vi "Configure Aperture.vi"(8 "error in (no error)":errorcluster, 9 "Aperture Time (1: 1s)":dbl(ring)=1.0 items=["1s"=1.0, "100ms"=0.1], 10 "Display (0: Primary Display)":i32(ring) items=["Primary Display", "Secondary Display"], 11 "VISA resource name":refnum<visa-resource-name>) -> (0 "error out":errorcluster, 3 "VISA resource name out":refnum<visa-resource-name>)   [LabVIEW 2020, in "Agilent 34405.lvlib"]
doc: "Configures the aperture time (also called gate time) for frequency measurements.\n\n<B>Notes:</B>\n(1) This VI affects the <B>Frequency</B> measurements only. \n(2) This VI only support <B>Agilent 34450A</B>."
uses:
  <instrlib>/Agilent 34405/Agilent 34405.lvlib
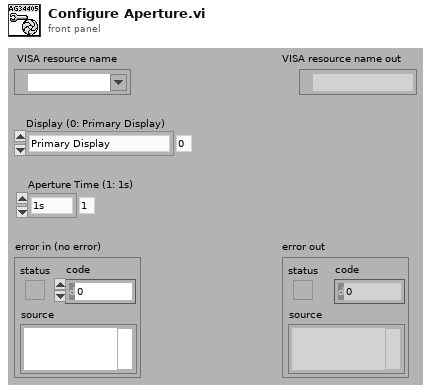
[diagram p1: front panel]
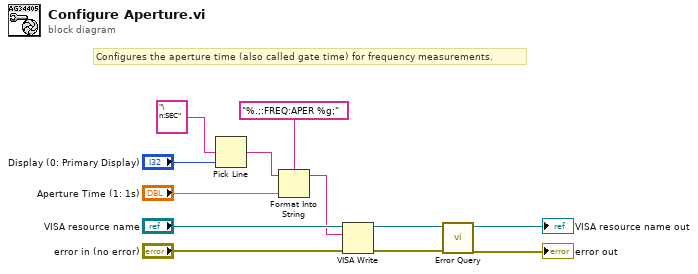
[diagram p0: block diagram]
diagram:
  # "Configures the aperture time (also called gate time) for frequency measurements."
  n1 = Pick Line(multi-line string="\n:SEC", line index="Display (0: Primary Display)") -> (output string=w1:string)  [unwired: 1 out]
  n2 = Format Into String(format string="%.;:FREQ:APER %g;", initial string=w1, "Aperture Time (1: 1s)") -> (resulting string=w3:string)  [unwired: 1 in, 1 out]
  n3 = VISA Write(VISA resource name="VISA resource name", write buffer=w3, error in (no error)="error in (no error)") -> (VISA resource name out=w10:refnum<visa-resource-name>, error out=w9:errorcluster)  [unwired: 1 out]
  n4 = call <instrlib>:"Error Query.vi"("error in (no error)"=w9, "VISA resource name"=w10) -> ("error out"=→"error out":errorcluster, "VISA resource name out"=→"VISA resource name out":refnum<visa-resource-name>)  [unwired: 8 out]
